vi "Split DMA by Direction and Ignore P2P.vi"() -> ()   [LabVIEW 2019]
uses:
  <vilib>/rvi/Emulation/niFpgaGetClockAttributes.vi
  <vilib>/rvi/Emulation/niFpgaSctlEmulationGetInTimedLoop.vi
  <vilib>/rvi/Emulation/niFpgaEmulationReportErrorSimple.vi
  <vilib>/rvi/Emulation/niFpgaCriticalErrorInLSC.vi
  <vilib>/rvi/interface/RandomDataEmulation/niFpgaRandomDataHandleErrors.vi
  <vilib>/rvi/DataTransferAndStorage/Container/XNode/niFpgaContainer.xnode
  <vilib>/rvi/interface/RandomDataEmulation/nirviRandomDataFpgaReadWriteTemplate.vi
  <vilib>/rvi/FIFO/Fifo_Resource/nirvififoEmulationP2P.vi
panel:
  out "Fast timeout 5":bool
  out "Fast timeout 4":bool
  out "Fast timeout 3":bool
  out "Fast timeout 2":bool
  in  "Group1.I16":i16
  in  "Group1.I8":i8
  in  "Group1.I64":i64
  in  "Group1.I32":i32
  in  "Group1.U16":u16
  in  "Group1.U8":u8
  in  "Group1.U64":u64
  in  "Group1.U32":u32
  in  "Group1.SGL":sgl
  in  "Group2.Boolean":bool
  out "Group1.I16 out":i16
  out "Group1.I8 out":i8
  out "Group1.I64 out":i64
  out "Group1.I32 out":i32
  out "Group1.U16 out":u16
  out "Group1.U8 out":u8
  out "Group1.U64 out":u64
  out "Group1.U32 out":u32
  out "Group1.SGL out":sgl
  out "Group2.Boolean out":bool
  in  "Group2.FXP24.5":fxp<+/-,24,5>
  in  "Group2.FXP16.5":fxp<+/-,16,5>
  in  "Group2.FXP32.8":fxp<+/-,32,8>
  in  "Group2.FXP64.32":fxp<+/-,64,32>
  out "Group2.FXP24.5 out":fxp<+/-,24,5>
  out "Group2.FXP16.5 out":fxp<+/-,16,5>
  out "Group2.FXP32.8 out":fxp<+/-,32,8>
  out "Group2.FXP64.32 out":fxp<+/-,64,32>
  in  "Group2.FXP16.7":fxp<+/-,16,7>
  out "Group2.FXP16.7 out":fxp<+/-,16,7>
  in  "Group2.FXP20.5":fxp<+/-,20,5>
  out "Group2.FXP20.5 out":fxp<+/-,20,5>
  in  "Group2.FXP27.5":fxp<+/-,27,5>
  out "Group2.FXP27.5 out":fxp<+/-,27,5>
  in  "Group2.FXP32.16":fxp<+/-,32,16>
  out "Group2.FXP32.16 out":fxp<+/-,32,16>
  in  "Group2.FXP16.3":fxp<+,16,3>
  out "Group2.FXP16.3 out":fxp<+,16,3>
  in  "Group2.FXP18.3":fxp<+,18,3>
  out "Group2.FXP18.3 out":fxp<+,18,3>
  in  "FXP18.3":fxp<+,18,3>
  out "FXP18.3 out":fxp<+,18,3>
  in  "FXP16.3":fxp<+,16,3>
  out "FXP16.3 out":fxp<+,16,3>
  in  "FXP32.16":fxp<+/-,32,16>
  out "FXP32.16 out":fxp<+/-,32,16>
  in  "FXP27.5":fxp<+/-,27,5>
  out "FXP27.5 out":fxp<+/-,27,5>
  in  "FXP20.5":fxp<+/-,20,5>
  out "FXP20.5 out":fxp<+/-,20,5>
  in  "FXP16.7":fxp<+/-,16,7>
  out "FXP16.7 out":fxp<+/-,16,7>
  out "FXP64.32 out":fxp<+/-,64,32>
  out "FXP32.8 out":fxp<+/-,32,8>
  out "FXP16.5 out":fxp<+/-,16,5>
  out "FXP24.5 out":fxp<+/-,24,5>
  in  "FXP64.32":fxp<+/-,64,32>
  in  "FXP32.8":fxp<+/-,32,8>
  in  "FXP16.5":fxp<+/-,16,5>
  in  "FXP24.5":fxp<+/-,24,5>
  out "Fast timeout":bool
  out "Med timeout":bool
  out "Slow timeout":bool
  in  "I16":i16
  in  "I8":i8
  in  "I64":i64
  in  "I32":i32
  in  "U16":u16
  in  "U8":u8
  in  "U64":u64
  in  "U32":u32
  in  "SGL":sgl
  in  "Boolean":bool
  out "I16 out":i16
  out "I8 out":i8
  out "I64 out":i64
  out "I32 out":i32
  out "U16 out":u16
  out "U8 out":u8
  out "U64 out":u64
  out "U32 out":u32
  out "SGL out":sgl
  out "Boolean out":bool
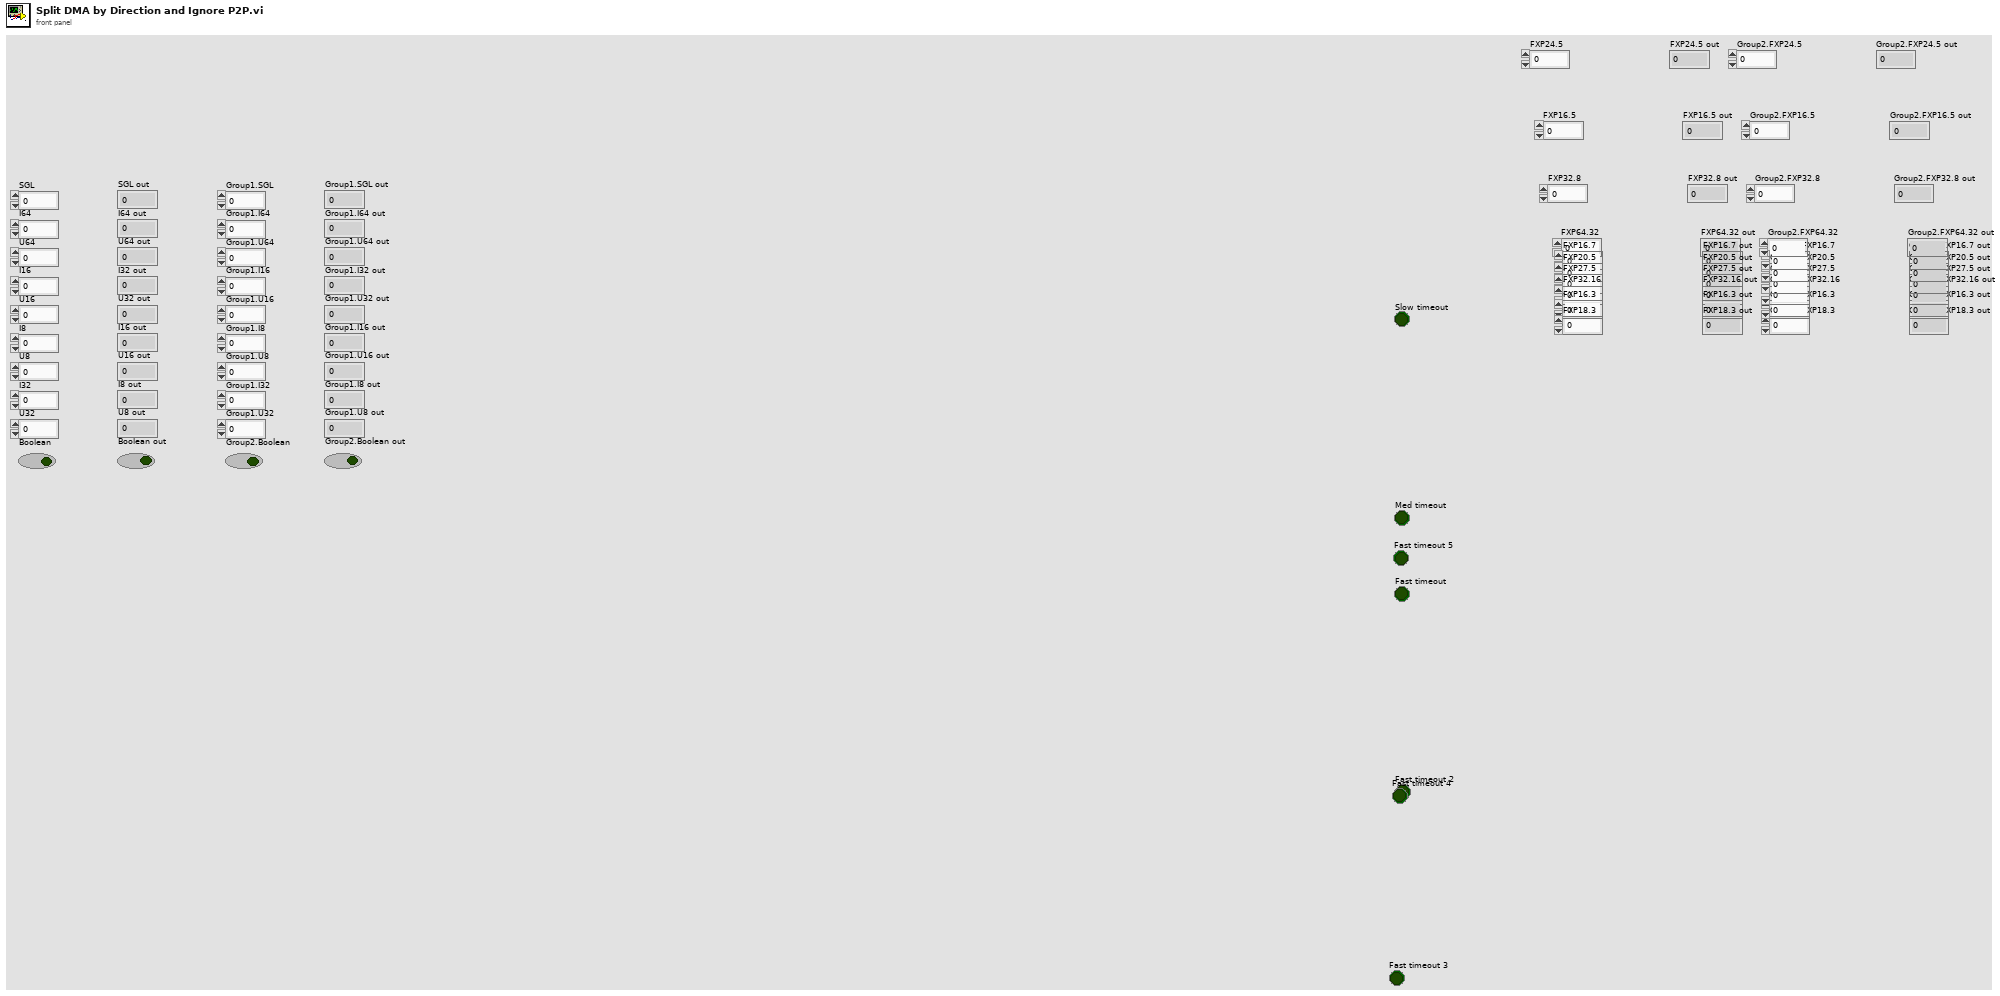
[diagram p1: front panel]
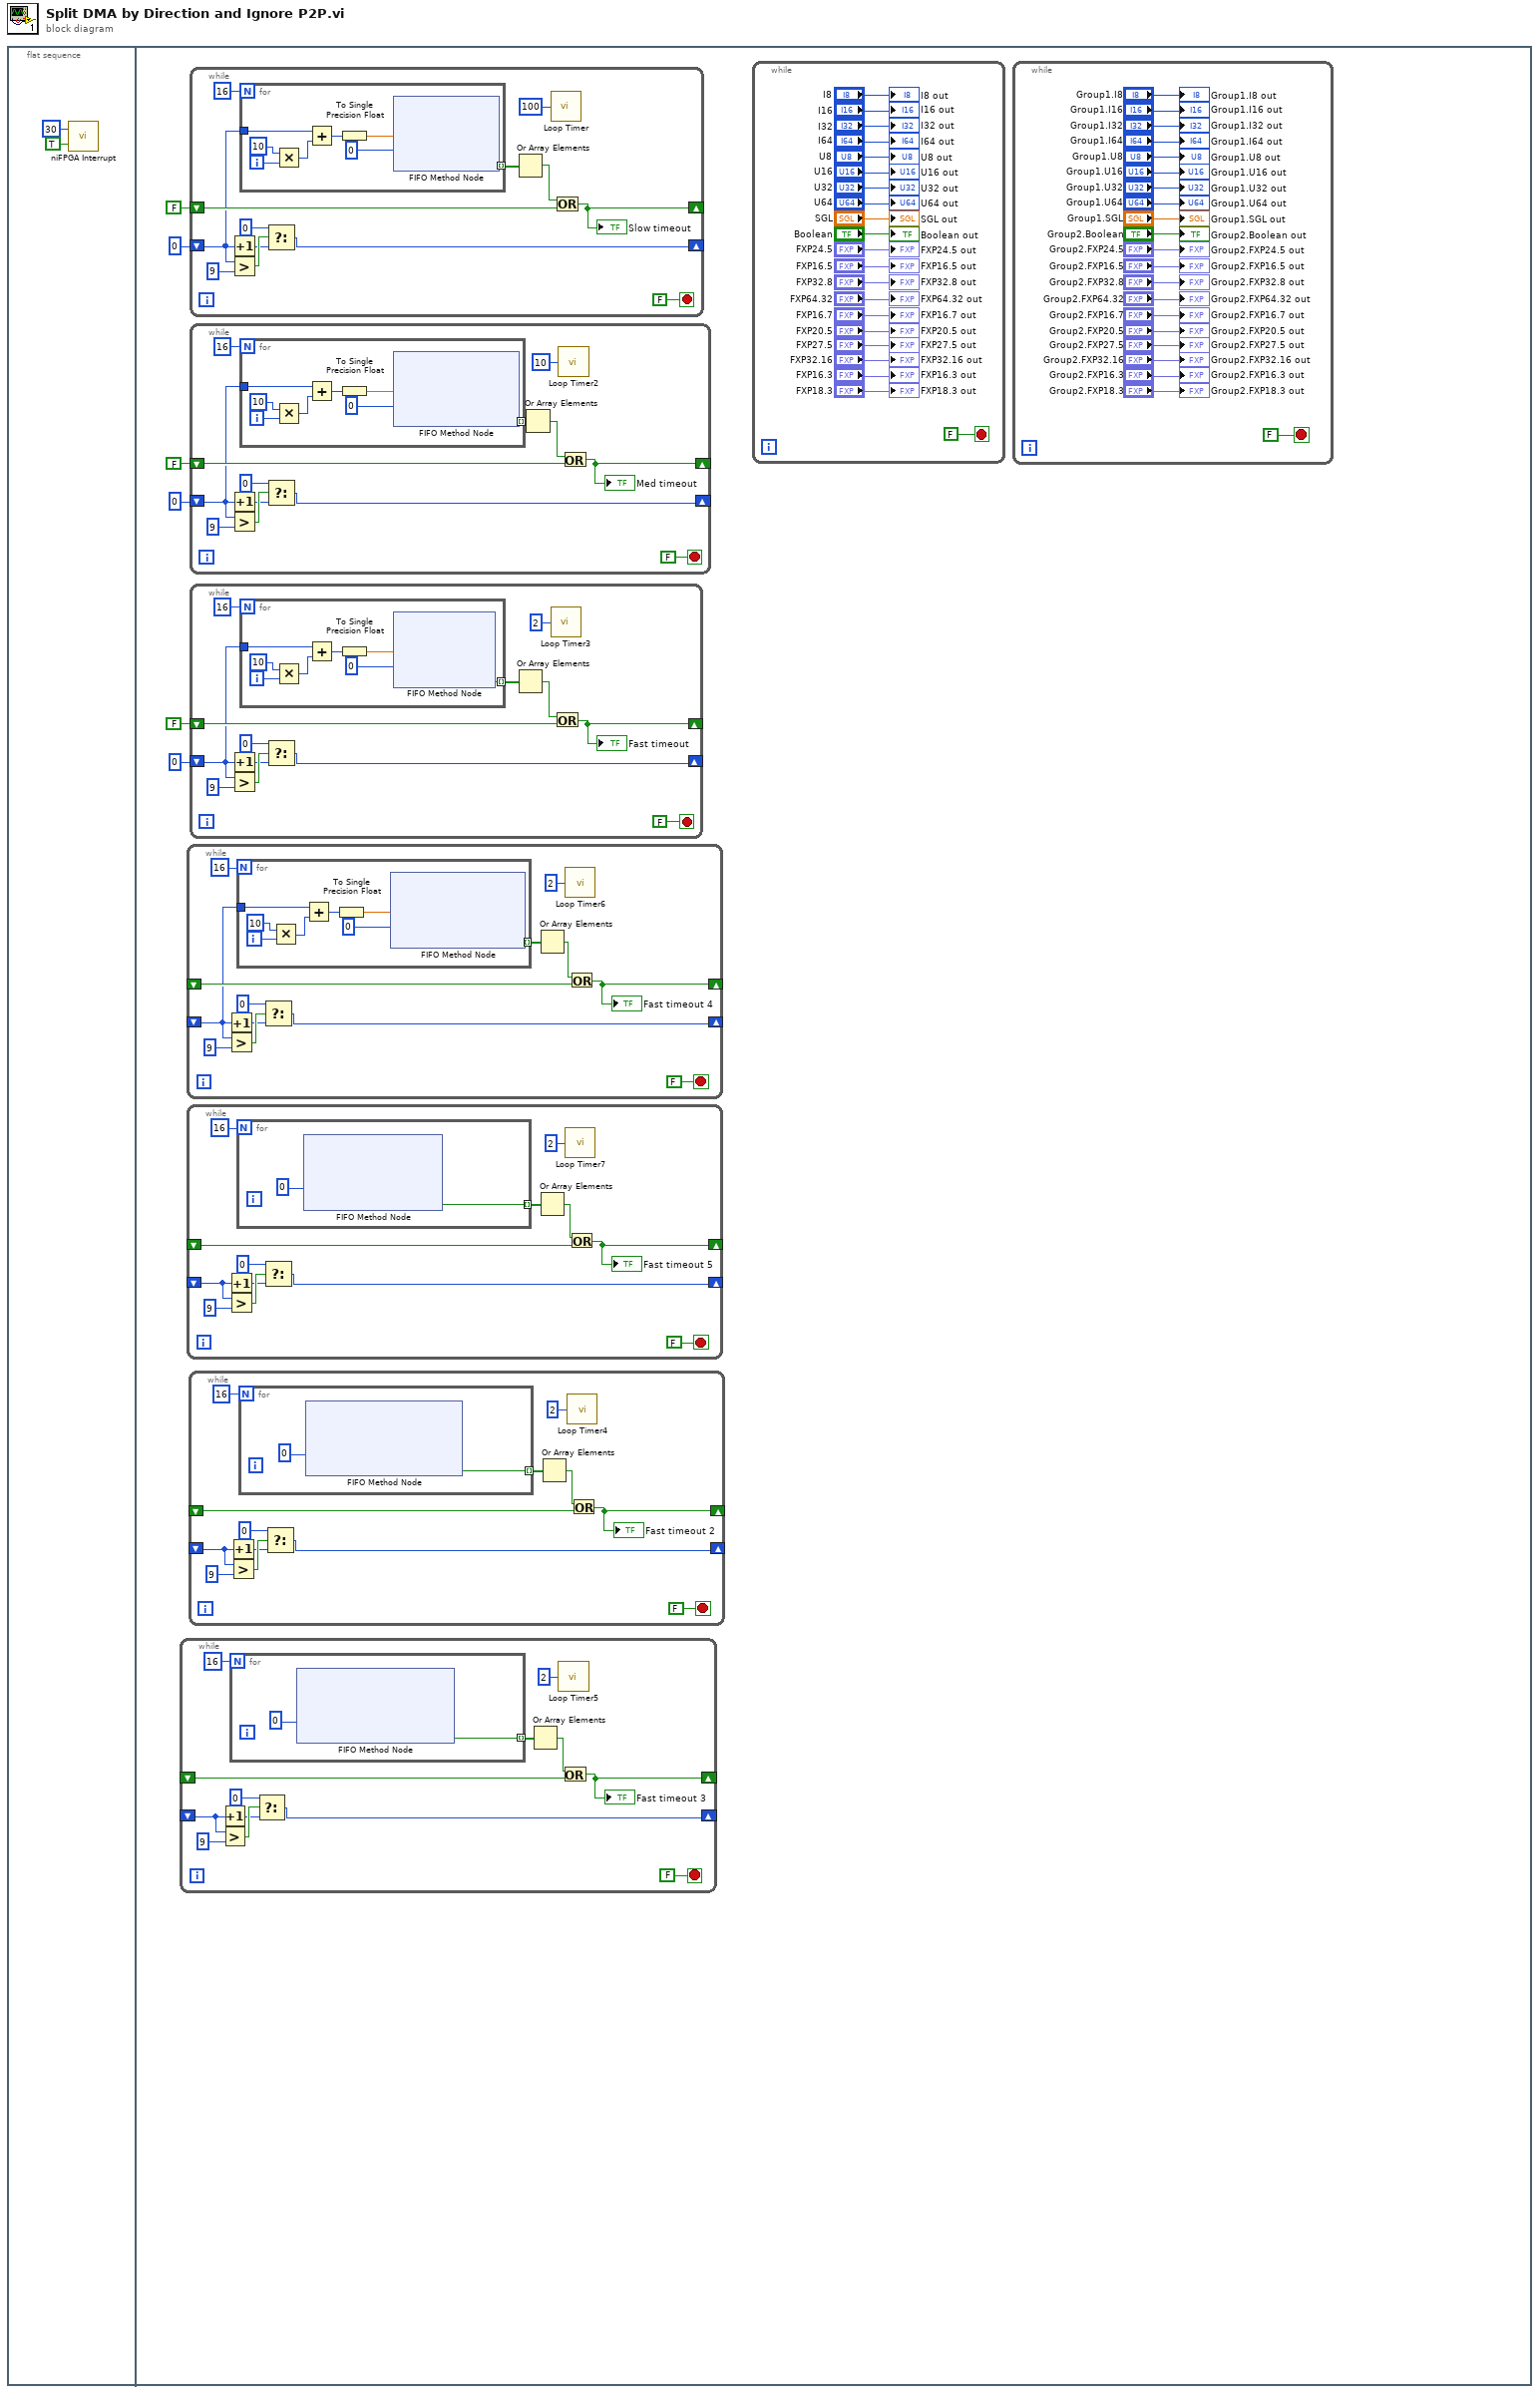
[diagram p0: block diagram]
diagram:
  n1 = flat-sequence {
    frame #0 {
      n2 = call <vilib>:"niFPGA Interrupt.vi"("Wait Until Cleared (F)"=TRUE, "IRQ Number (0)"=u8 30) -> ()  [unwired: 1 in]
    }
    frame #1 {
      n3 = while {
        shift-right: [w157] -> _
        shift-left: _ -> [w151]
        shift-right: [w152] -> _
        shift-left: _ -> [w153]
        stop <- FALSE stop-if-true
        n4 = Increment(x=w151) -> (x+1=w155:i32)
        n5 = Greater?(x=w151, y=9) -> (0:w161:bool)
        n6 = for {
          N: 16 -> [_]
          tunnel: [w163] -> w150 mode=indexing
          n7 = xnode ("FIFO Method Node")("Timeout"=0) -> ("Timed Out?"=w163:bool)  [unwired: 1 in, 2 out]
        }
        n8 = Select(t=0, s=w161, f=w155) -> (s? t:f=w157:i32)
        n9 = Or Array Elements(Boolean array=w150) -> (logical OR=w154:bool)
        n10 = call "Loop Timer5"("Count(uSec)"=u32 2) -> ()  [unwired: 1 out]
        n11 = Or(x=w154, y=w153) -> (x .or. y?=w152:bool)
        "Fast timeout 3" <- w152
      }
      n12 = while {
        shift-right: [w31] -> _
        shift-left: _ -> [w24]
        shift-right: [w25] -> _
        shift-left: _ -> [w26]
        stop <- FALSE stop-if-true
        n13 = Increment(x=w24) -> (x+1=w29:i32)
        n14 = Greater?(x=w24, y=9) -> (0:w35:bool)
        n15 = for {
          N: 16 -> [_]
          tunnel: w24 -> [w44]
          tunnel: [w37] -> w28 mode=indexing
          i -> [w43]
          n16 = Multiply(x=10, y=w43) -> (x*y=w41:i32)
          n17 = Add(x=w44, y=w41) -> (x+y=w40:i32)
          n18 = To Single Precision Float(number=w40) -> (single precision float=w39:sgl)
          n19 = xnode ("FIFO Method Node")("Element"=w39, "Timeout"=0) -> ("Timed Out?"=w37:bool)  [unwired: 1 in, 1 out]
        }
        n20 = Select(t=0, s=w35, f=w29) -> (s? t:f=w31:i32)
        n21 = Or Array Elements(Boolean array=w28) -> (logical OR=w27:bool)
        n22 = call "Loop Timer6"("Count(uSec)"=u32 2) -> ()  [unwired: 1 out]
        n23 = Or(x=w27, y=w26) -> (x .or. y?=w25:bool)
        "Fast timeout 4" <- w25
      }
      n24 = while {
        shift-right: [w16] -> _
        shift-left: _ -> [w10]
        shift-right: [w11] -> _
        shift-left: _ -> [w12]
        stop <- FALSE stop-if-true
        n25 = Increment(x=w10) -> (x+1=w14:i32)
        n26 = Greater?(x=w10, y=9) -> (0:w20:bool)
        n27 = for {
          N: 16 -> [_]
          tunnel: [w22] -> w9 mode=indexing
          n28 = xnode ("FIFO Method Node")("Timeout"=0) -> ("Timed Out?"=w22:bool)  [unwired: 1 in, 2 out]
        }
        n29 = Select(t=0, s=w20, f=w14) -> (s? t:f=w16:i32)
        n30 = Or Array Elements(Boolean array=w9) -> (logical OR=w13:bool)
        n31 = call "Loop Timer7"("Count(uSec)"=u32 2) -> ()  [unwired: 1 out]
        n32 = Or(x=w13, y=w12) -> (x .or. y?=w11:bool)
        "Fast timeout 5" <- w11
      }
      n33 = while {
        shift-right: [w172] -> _
        shift-left: _ -> [w166]
        shift-right: [w167] -> _
        shift-left: _ -> [w168]
        stop <- FALSE stop-if-true
        n34 = Increment(x=w166) -> (x+1=w170:i32)
        n35 = Greater?(x=w166, y=9) -> (0:w176:bool)
        n36 = for {
          N: 16 -> [_]
          tunnel: [w178] -> w165 mode=indexing
          n37 = xnode ("FIFO Method Node")("Timeout"=0) -> ("Timed Out?"=w178:bool)  [unwired: 1 in, 2 out]
        }
        n38 = Select(t=0, s=w176, f=w170) -> (s? t:f=w172:i32)
        n39 = Or Array Elements(Boolean array=w165) -> (logical OR=w169:bool)
        n40 = call "Loop Timer4"("Count(uSec)"=u32 2) -> ()  [unwired: 1 out]
        n41 = Or(x=w169, y=w168) -> (x .or. y?=w167:bool)
        "Fast timeout 2" <- w167
      }
      n42 = while {
        shift-right: [w115] -> _
        shift-left: 0 ("t") -> [w108]
        shift-right: [w109] -> _
        shift-left: FALSE -> [w110]
        stop <- FALSE stop-if-true
        n43 = Increment(x=w108) -> (x+1=w113:i32)
        n44 = Greater?(x=w108, y=9) -> (0:w119:bool)
        n45 = for {
          N: 16 -> [_]
          tunnel: w108 -> [w128]
          tunnel: [w121] -> w112 mode=indexing
          i -> [w127]
          n46 = Multiply(x=10, y=w127) -> (x*y=w125:i32)
          n47 = Add(x=w128, y=w125) -> (x+y=w124:i32)
          n48 = To Single Precision Float(number=w124) -> (single precision float=w123:sgl)
          n49 = xnode ("FIFO Method Node")("Element"=w123, "Timeout"=0) -> ("Timed Out?"=w121:bool)  [unwired: 1 in, 1 out]
        }
        n50 = Select(t=0, s=w119, f=w113) -> (s? t:f=w115:i32)
        n51 = Or Array Elements(Boolean array=w112) -> (logical OR=w111:bool)
        n52 = call "Loop Timer"("Count(uSec)"=u32 100) -> ()  [unwired: 1 out]
        n53 = Or(x=w111, y=w110) -> (x .or. y?=w109:bool)
        "Slow timeout" <- w109
      }
      n54 = while {
        shift-right: [w94] -> _
        shift-left: 0 ("t") -> [w87]
        shift-right: [w88] -> _
        shift-left: FALSE -> [w89]
        stop <- FALSE stop-if-true
        n55 = Increment(x=w87) -> (x+1=w92:i32)
        n56 = Greater?(x=w87, y=9) -> (0:w98:bool)
        n57 = for {
          N: 16 -> [_]
          tunnel: w87 -> [w107]
          tunnel: [w100] -> w91 mode=indexing
          i -> [w106]
          n58 = Multiply(x=10, y=w106) -> (x*y=w104:i32)
          n59 = Add(x=w107, y=w104) -> (x+y=w103:i32)
          n60 = To Single Precision Float(number=w103) -> (single precision float=w102:sgl)
          n61 = xnode ("FIFO Method Node")("Element"=w102, "Timeout"=0) -> ("Timed Out?"=w100:bool)  [unwired: 1 in, 1 out]
        }
        n62 = Select(t=0, s=w98, f=w92) -> (s? t:f=w94:i32)
        n63 = Or Array Elements(Boolean array=w91) -> (logical OR=w90:bool)
        n64 = call "Loop Timer2"("Count(uSec)"=u32 10) -> ()  [unwired: 1 out]
        n65 = Or(x=w90, y=w89) -> (x .or. y?=w88:bool)
        "Med timeout" <- w88
      }
      n66 = while {
        shift-right: [w73] -> _
        shift-left: 0 ("t") -> [w66]
        shift-right: [w67] -> _
        shift-left: FALSE -> [w68]
        stop <- FALSE stop-if-true
        n67 = Increment(x=w66) -> (x+1=w71:i32)
        n68 = Greater?(x=w66, y=9) -> (0:w77:bool)
        n69 = for {
          N: 16 -> [_]
          tunnel: w66 -> [w86]
          tunnel: [w79] -> w70 mode=indexing
          i -> [w85]
          n70 = Multiply(x=10, y=w85) -> (x*y=w83:i32)
          n71 = Add(x=w86, y=w83) -> (x+y=w82:i32)
          n72 = To Single Precision Float(number=w82) -> (single precision float=w81:sgl)
          n73 = xnode ("FIFO Method Node")("Element"=w81, "Timeout"=0) -> ("Timed Out?"=w79:bool)  [unwired: 1 in, 1 out]
        }
        n74 = Select(t=0, s=w77, f=w71) -> (s? t:f=w73:i32)
        n75 = Or Array Elements(Boolean array=w70) -> (logical OR=w69:bool)
        n76 = call "Loop Timer3"("Count(uSec)"=u32 2) -> ()  [unwired: 1 out]
        n77 = Or(x=w69, y=w68) -> (x .or. y?=w67:bool)
        "Fast timeout" <- w67
      }
      n78 = while {
        stop <- FALSE stop-if-true
        "I16 out" <- "I16"
        "I8 out" <- "I8"
        "I64 out" <- "I64"
        "I32 out" <- "I32"
        "U16 out" <- "U16"
        "U8 out" <- "U8"
        "U64 out" <- "U64"
        "U32 out" <- "U32"
        "SGL out" <- "SGL"
        "Boolean out" <- "Boolean"
        "FXP24.5 out" <- "FXP24.5"
        "FXP16.5 out" <- "FXP16.5"
        "FXP32.8 out" <- "FXP32.8"
        "FXP64.32 out" <- "FXP64.32"
        "FXP16.7 out" <- "FXP16.7"
        "FXP20.5 out" <- "FXP20.5"
        "FXP27.5 out" <- "FXP27.5"
        "FXP32.16 out" <- "FXP32.16"
        "FXP16.3 out" <- "FXP16.3"
        "FXP18.3 out" <- "FXP18.3"
      }
      n79 = while {
        stop <- FALSE stop-if-true
        "Group1.I16 out" <- "Group1.I16"
        "Group1.I8 out" <- "Group1.I8"
        "Group1.I64 out" <- "Group1.I64"
        "Group1.I32 out" <- "Group1.I32"
        "Group1.U16 out" <- "Group1.U16"
        "Group1.U8 out" <- "Group1.U8"
        "Group1.U64 out" <- "Group1.U64"
        "Group1.U32 out" <- "Group1.U32"
        "Group1.SGL out" <- "Group1.SGL"
        "Group2.Boolean out" <- "Group2.Boolean"
        "Group2.FXP24.5 out" <- "Group2.FXP24.5"
        "Group2.FXP16.5 out" <- "Group2.FXP16.5"
        "Group2.FXP32.8 out" <- "Group2.FXP32.8"
        "Group2.FXP64.32 out" <- "Group2.FXP64.32"
        "Group2.FXP16.7 out" <- "Group2.FXP16.7"
        "Group2.FXP20.5 out" <- "Group2.FXP20.5"
        "Group2.FXP27.5 out" <- "Group2.FXP27.5"
        "Group2.FXP32.16 out" <- "Group2.FXP32.16"
        "Group2.FXP16.3 out" <- "Group2.FXP16.3"
        "Group2.FXP18.3 out" <- "Group2.FXP18.3"
      }
    }
  }
